vi "Process.vi"(8 "error in":errorcluster, 11 "MauiTemplate":refnum<class "SMO.UI.MAUI.Basic.lvclass">) -> (0 "error out":errorcluster, 3 "MauiTemplate out":refnum<class "SMO.UI.MAUI.Basic.lvclass">)   [LabVIEW 2016, in "SMO.UI.MAUI.Basic.lvclass"]
doc: "---------------------------------------------------------------\nJKI State Machine Objects™\nhttp://jki.net/state-machine-objects/\nCopyright (C) 2005-2015, JKI <info@jki.net>\nALL RIGHTS RESERVED"
uses:
  SMO.UI.MAUI.Basic.lvclass
  C:/Program Files (x86)/National Instruments/LabVIEW 2016/vi.lib/JKI/JKI SMO/SMO/SMO.lvclass
  C:/Program Files (x86)/National Instruments/LabVIEW 2016/vi.lib/Levylab/SMO.UI.MAUI/SMO.UI.MAUI.lvclass
  C:/Program Files (x86)/National Instruments/LabVIEW 2016/vi.lib/JKI/JKI SMO/SMO.UI/SMO.UI.lvclass
  <vilib>/JKI/JKI SMO/SMO/Typedefs/Parent Call--Enum.ctl
  <vilib>/Levylab/SMO.UI.MAUI/Typedefs/PanelData.ctl
  <vilib>/Levylab/SMO.UI.MAUI/SMO.UI.MAUI.lvclass
  <vilib>/JKI/JKI SMO/SMO/SMO.lvclass
  <vilib>/JKI/JKI SMO/SMO.UI/SMO.UI.lvclass
panel:
  out "Title":string
  in  "PopLeft":bool
  in  "PopRight":bool
  in  "Right Ring":u16(ring)
  in  "Left Ring":u16(ring)
  # "For instructions on how to use the JKI State Machine Objects, examples and video tutorials, visit:\nhttp://jki.net/state-machine-objects/\n\nJKI State Machine Objects™\nhttp://jki.net/state-machine-objects/\nCopyright (C) 2005-2015, JKI <info@jki.net>\nALL RIGHTS RESERVED"
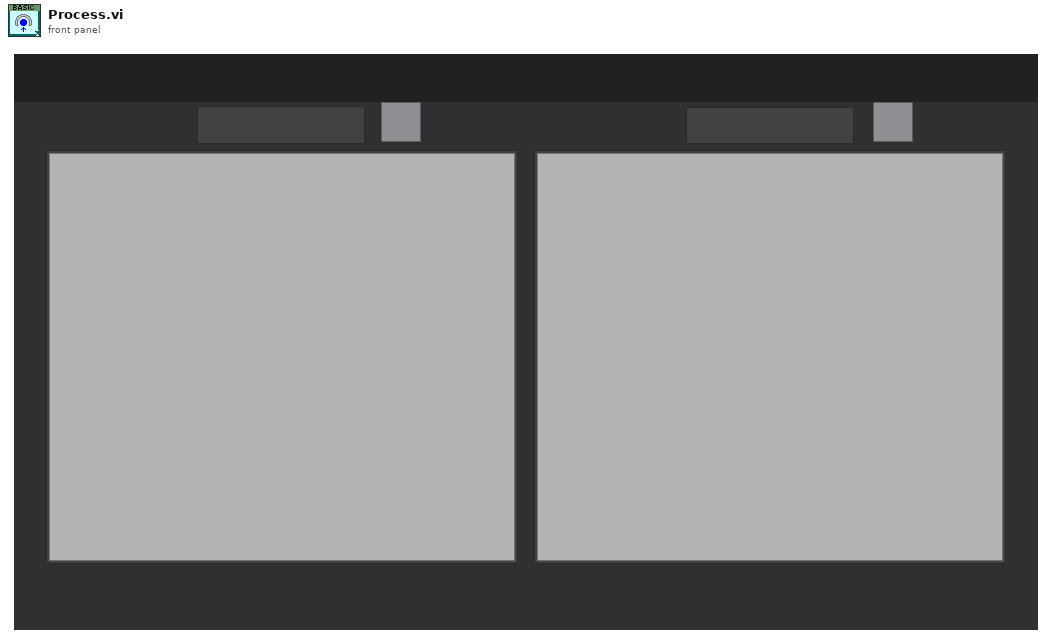
[diagram p1: front panel]
types:
  T1 = typedef "SMO.lvclass/Parent Call--Enum.ctl" = enum16{"Allows parent to run", "Does not request parent to run"}
  T2 = enum32{"invalid app kind", "Development System", "Run Time System", "Student Edition", "Embedded LabVIEW", "Evaluation", "Custom"}
  T3 = enum32{"Invalid", "Standard", "Closed", "Hidden", "Minimized", "Maximized"}
  T4 = enum32{"Bad", "Idle", "Run top level", "Running"}
  T5 = cluster{"Core":cluster{"Current VI Reference":refnum<vi>, "Close Panel on Exit?":bool, "error":errorcluster}, "MAUI":cluster{"Active Index":i32, "Panel Index":i32, "Pop Index":i32}, "Self Reference":refnum<class "SMO.UI.MAUI.Basic.lvclass">}
  T6 = cluster{"Active Index":i32, "Panel Index":i32, "Pop Index":i32}
  T7 = cluster{"Current VI Reference":refnum<vi>, "Close Panel on Exit?":bool, "error":errorcluster}
  T8 = typedef "SMO.lvclass/Protected Events.ctl" = cluster{"StopProcesses":refnum<user-event>, "AbortProcesses":refnum<user-event>, "Config Changed":refnum<user-event>, "Dependency":refnum<user-event>}
  T9 = typedef "SMO.UI.MAUI.lvclass/PublicEvents--Cluster.ctl" = cluster{"ReadyForInfo ":refnum<user-event>}
  T10 = typedef "SMO.UI.MAUI.lvclass/PanelData.ctl" = cluster{"SubPanel":refnum<vi>, "Ring":refnum<vi>, "Active":i32}
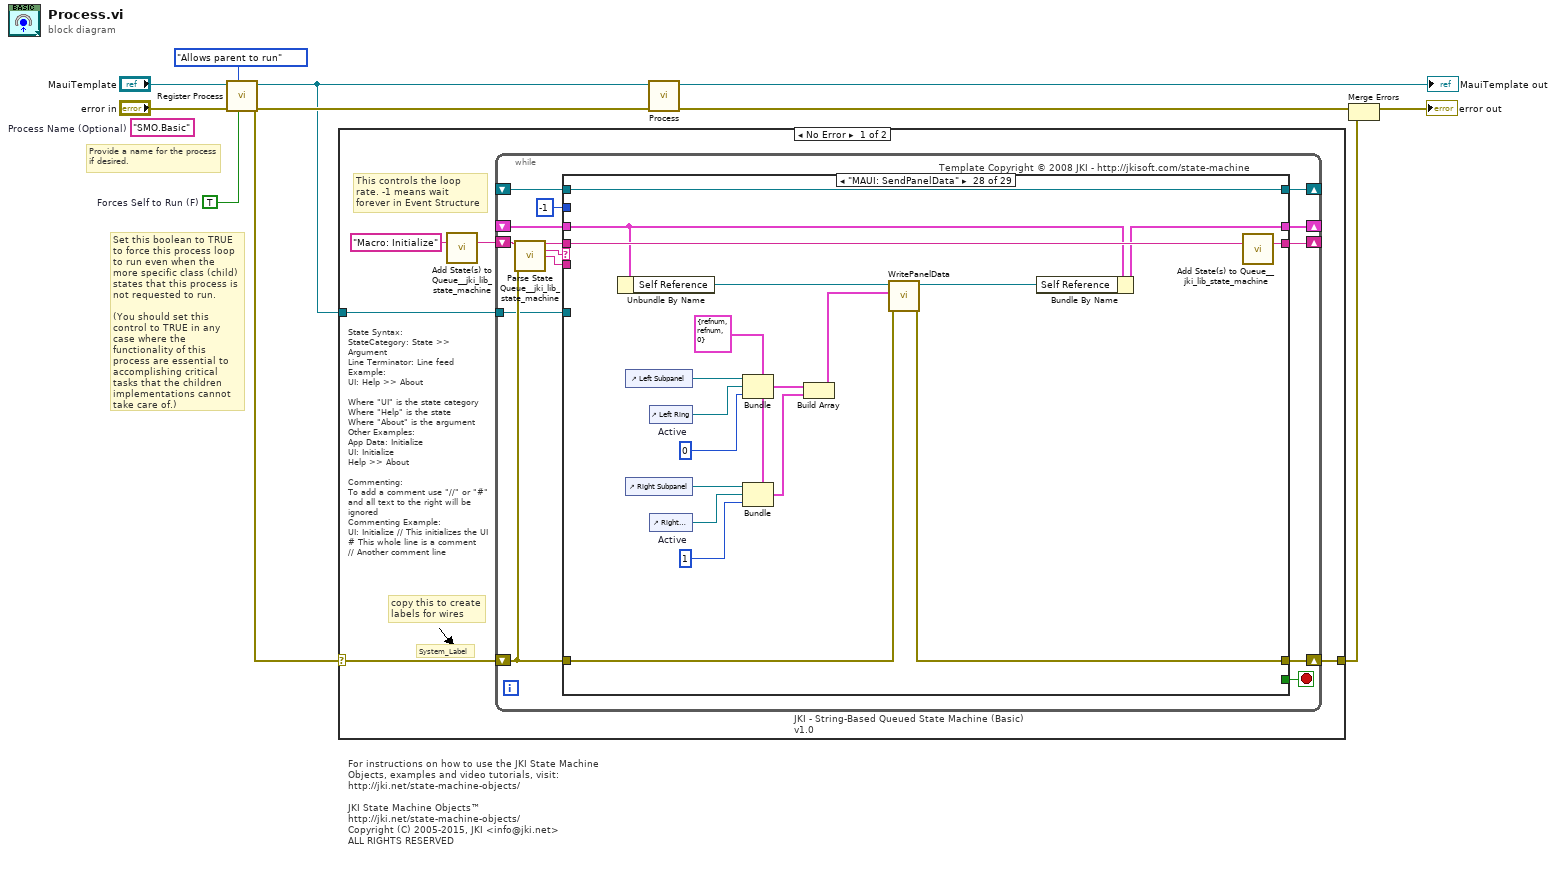
[diagram p0: block diagram]
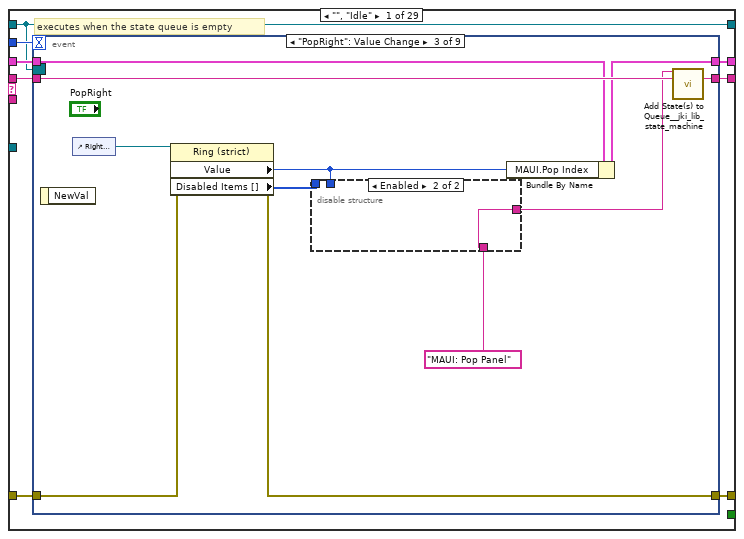
[diagram p2: hidden frame]
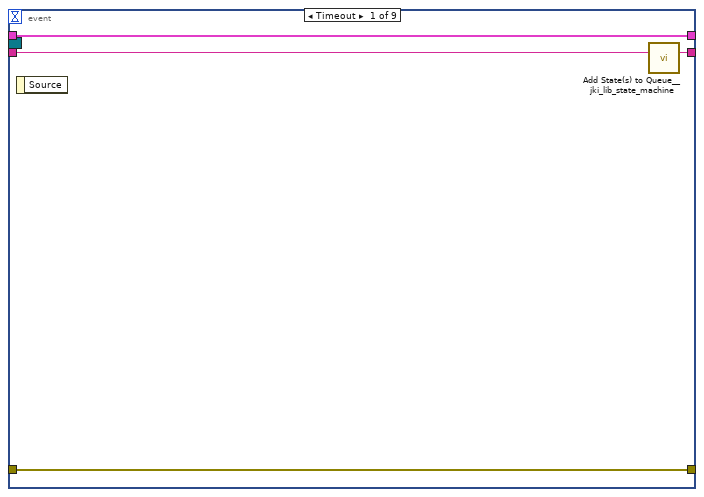
[diagram p3: hidden frame]
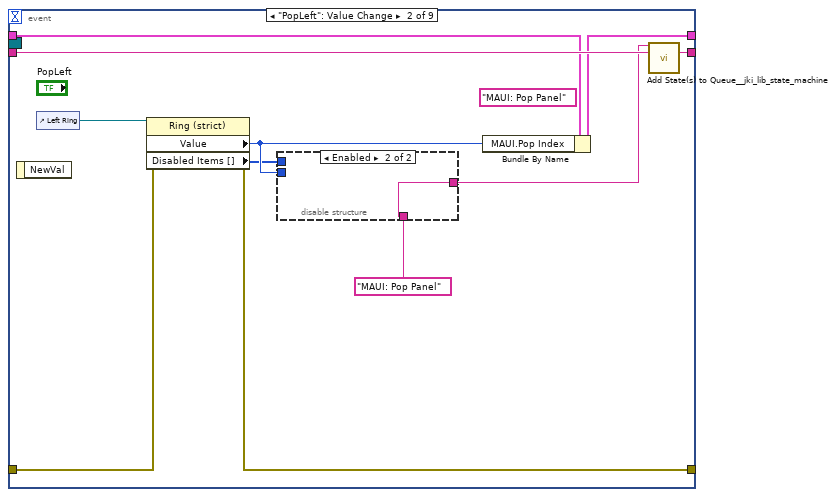
[diagram p4: hidden frame]
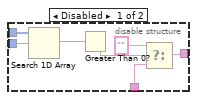
[diagram p5: hidden frame]
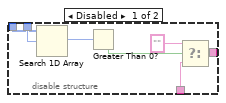
[diagram p6: hidden frame]
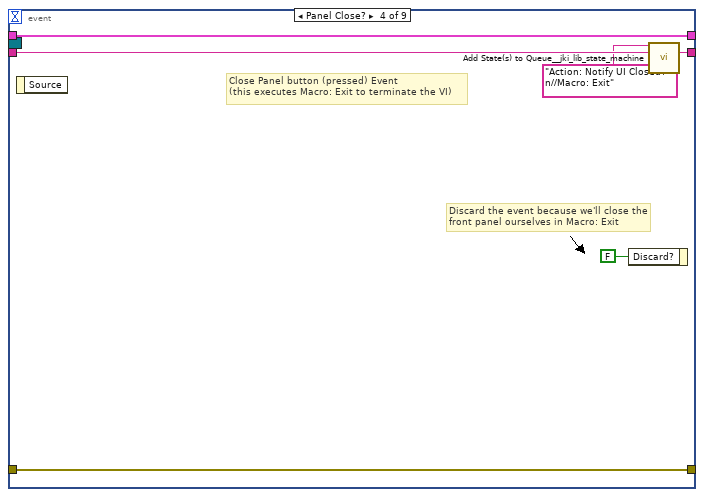
[diagram p7: hidden frame]
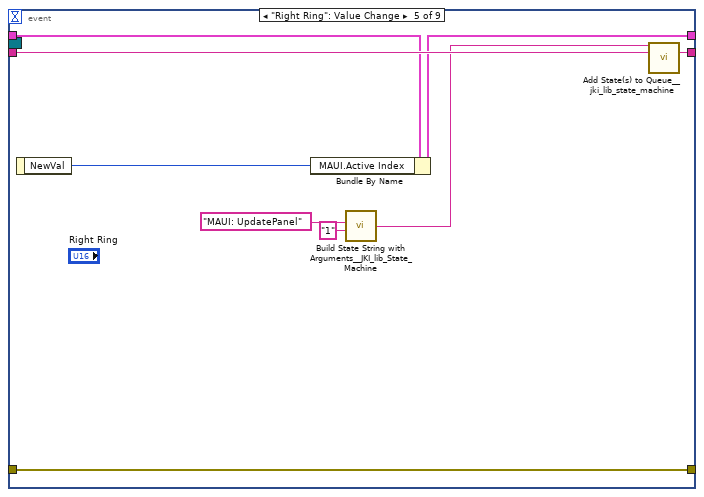
[diagram p8: hidden frame]
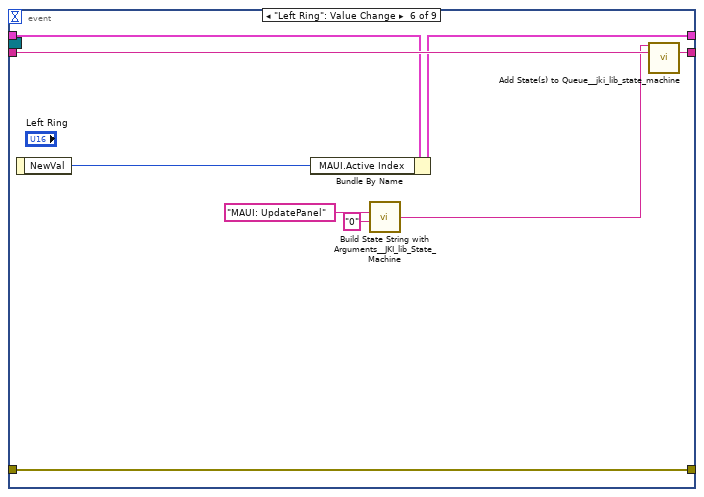
[diagram p9: hidden frame]
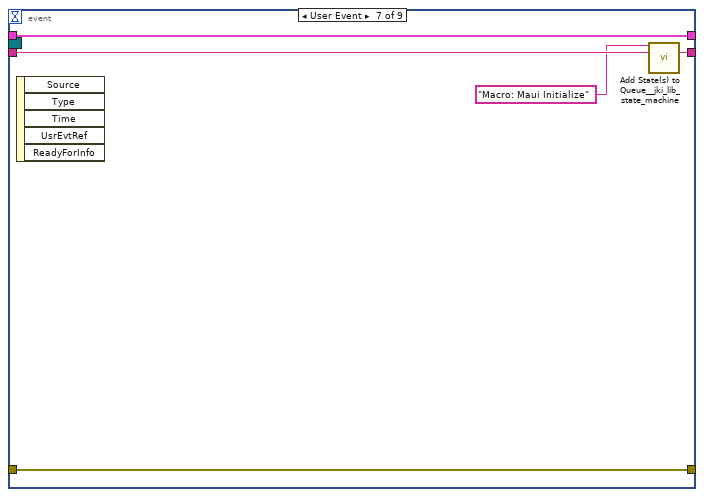
[diagram p10: hidden frame]
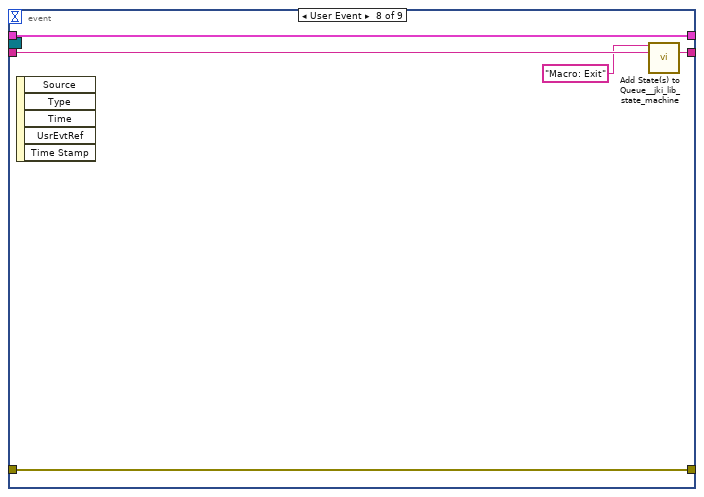
[diagram p11: hidden frame]
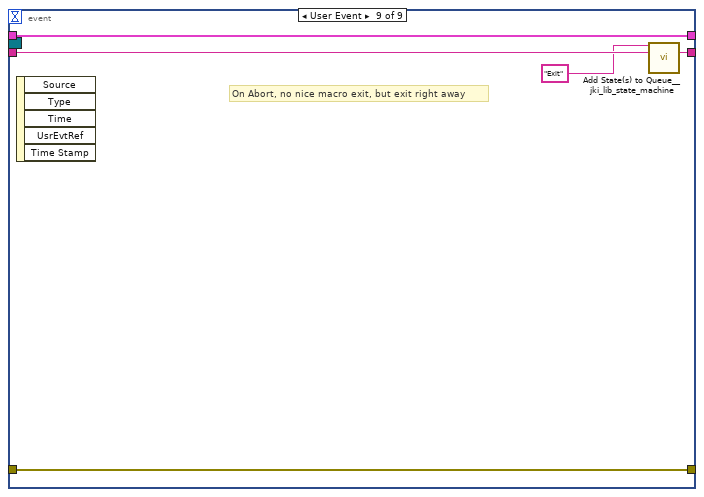
[diagram p12: hidden frame]
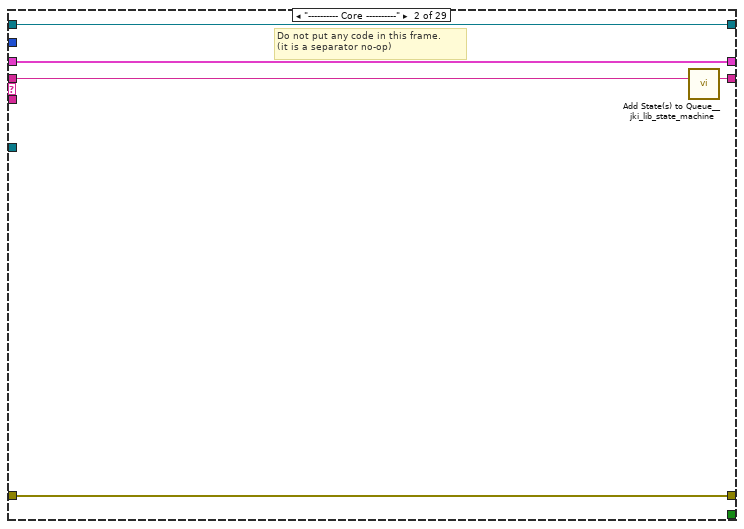
[diagram p13: hidden frame]
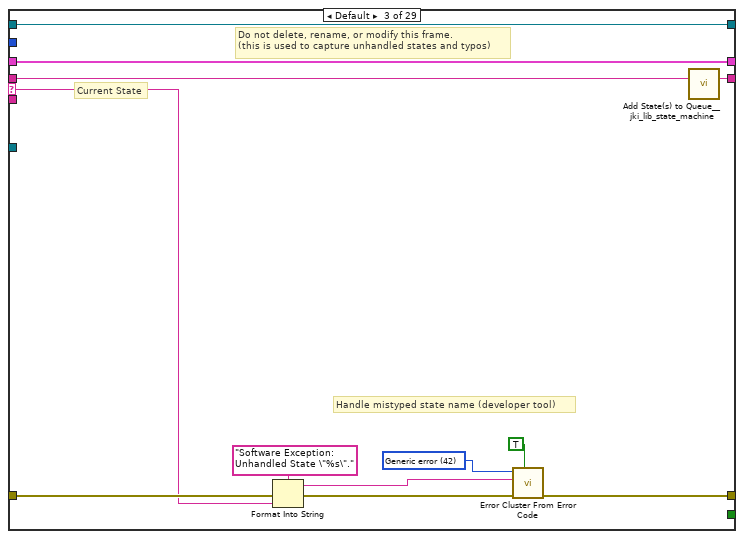
[diagram p14: hidden frame]
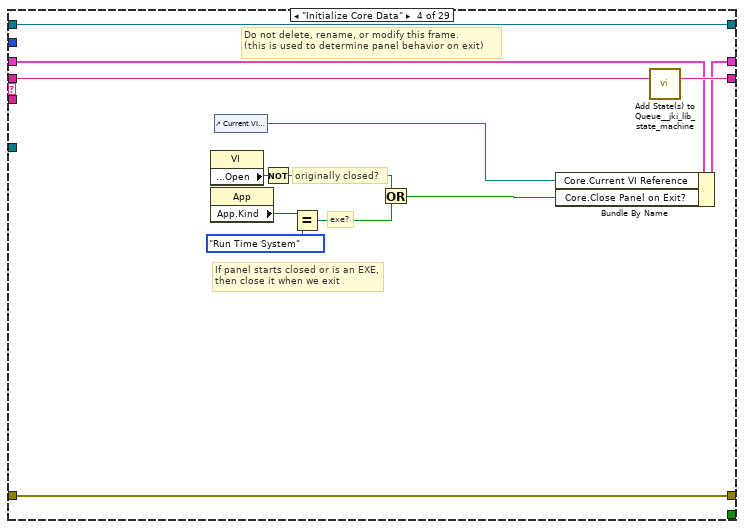
[diagram p15: hidden frame]
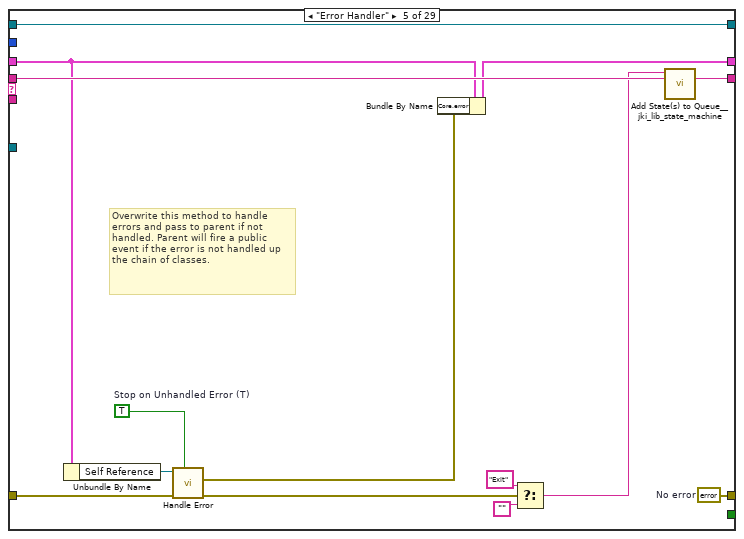
[diagram p16: hidden frame]
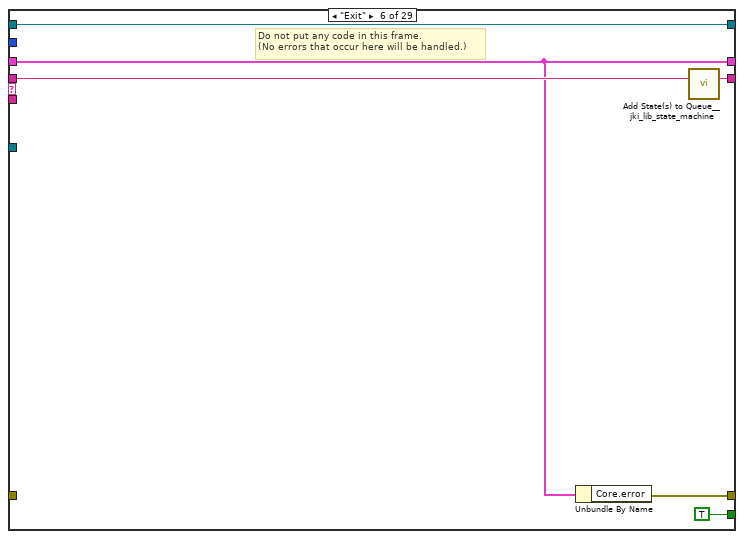
[diagram p17: hidden frame]
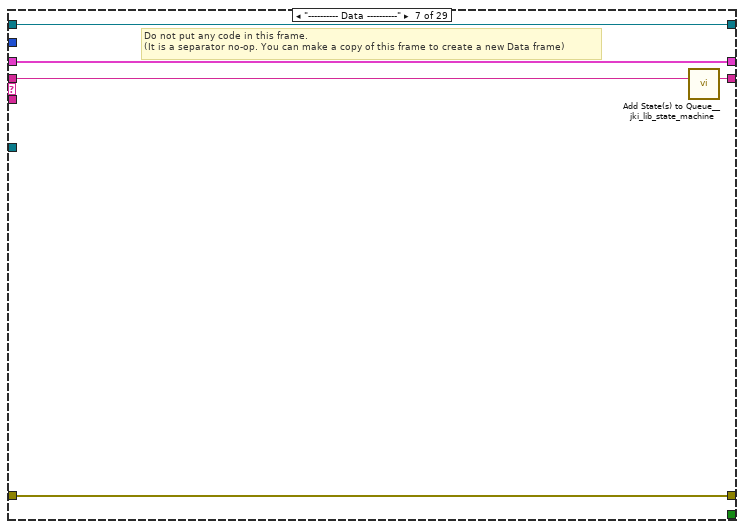
[diagram p18: hidden frame]
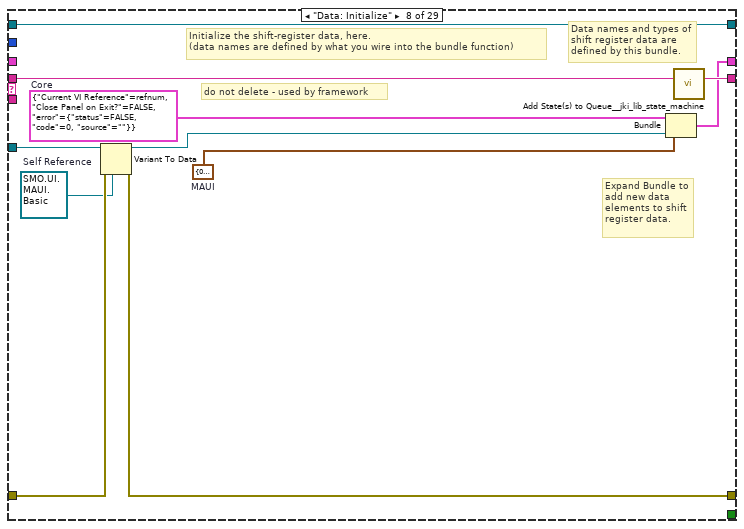
[diagram p19: hidden frame]
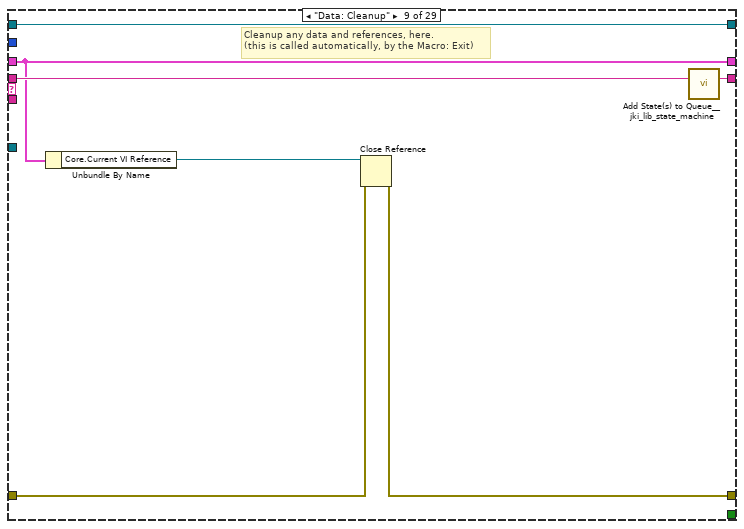
[diagram p20: hidden frame]
diagram:
  w2 = TRUE  # Forces Self to Run (F)
  (unwired) "SMO.Basic"  # Process Name (Optional)
  # "Provide a name for the process\nif desired."
  # "Set this boolean to TRUE to force this process loop to run even when the more specific class (child) states that this process is not requested to run.\n\n(You should set this control to TRUE in any case where the functionality of this process are essential to accomplishing critical tasks that the children implementations cannot take care of.)"
  # "For instructions on how to use the JKI State Machine Objects, examples and video tutorials, visit:\nhttp://jki.net/state-machine-objects/\n\nJKI State Machine Objects™\nhttp://jki.net/state-machine-objects/\nCopyright (C) 2005-2015, JKI <info@jki.net>\nALL RIGHTS RESERVED"
  n1 = call <vilib>:"Register Process.vi"("Forces Self to Run (F)"=w2, "Parent Call"=Parent_Call--Enum."Allows parent to run", "error in (no error)"="error in", "SMO"="MauiTemplate") -> ("error out"=w7:errorcluster, "SMO out"=w1:refnum<class "SMO.UI.MAUI.Basic.lvclass">)  [unwired: 6 in]
  n2 = case shown="No Error" w7 {
    selector: w7 -> [w12 w408]
    tunnel: w1 -> [w13 _]
    tunnel: [w11 w408] -> w4
    frame No Error {
      # "State Syntax:\nStateCategory: State >> Argument\nLine Terminator: Line feed\nExample:\nUI: Help >> About\n\nWhere \"UI\" is the state category\nWhere \"Help\" is the state\nWhere \"About\" is the argument\nOther Examples:\nApp Data: Initialize\nUI: Initialize\nHelp >> About\n\nCommenting:\nTo add a comment use \"//\" or \"#\" and all text to the right will be ignored\nCommenting Example:\nUI: Initialize // This initializes the UI\n# This whole line is a comment\n// Another comment line"
      # "copy this to create labels for wires"
      # "This controls the loop rate. -1 means wait forever in Event Structure"
      # "System_Label"
      n3 = call <vilib>:"Add State(s) to Queue__jki_lib_state_machine.vi"("State(s) in (\"\")"="Macro: Initialize") -> ("States Out"=w15:string)  [unwired: 14 in]
      n4 = while "JKI - String-Based Queued State Machine (Basic) v1.0" {
        shift-right: [w22] -> _
        shift-left: _ -> [w21]
        shift-right: [w25] -> w11
        shift-left: w12 -> [w19]
        shift-right: [w24] -> _
        shift-left: w15 -> [w26]
        tunnel: w13 -> [w18]
        shift-right: [w17] -> _
        shift-left: _ -> [w16]
        stop <- w23 stop-if-true
        # "Template Copyright © 2008 JKI - http://jkisoft.com/state-machine"
        n5 = call <vilib>:"Parse State Queue__jki_lib_state_machine.vi"("State Queue"=w26, "Error In (no error)"=w19) -> ("Remaining States"=w28:string, "Current State"=w29:string, "Arguments"=w27:string)  [unwired: 11 in]
        n6 = case shown="\"MAUI: SendPanelData\"" w29 {
          selector: w29 -> [_ _ w125 _ _ _ _ _ _ _ _ _ _ _ _ _ _ _ _ _ _ _ _ _ _ _ _ _ _]
          tunnel: w28 -> [w37 w123 w129 w148 w162 w168 w173 w184 w191 w196 w214 w221 w237 w269 w283 w289 w303 w308 w319 w324 w336 w342 w347 w354 w361 w366 w376 w395 w407]
          tunnel: w27 -> [_ _ _ _ _ _ _ _ _ _ _ w215 w231 _ _ _ _ _ _ _ _ _ _ _ _ _ _ _ w402]
          tunnel: w21 -> [w35 w120 w127 w139 w156 w164 w170 _ w186 w193 w209 w219 w233 w266 w279 w286 w294 w305 w316 w321 w334 w340 w345 w351 w357 w364 w371 w392 w404]
          tunnel: [w34 w121 w131 w145 w157 w163 w171 w180 w187 w194 w198 w216 w234 w267 w281 w287 w301 w306 w310 w322 w330 w338 w343 w348 w358 w362 w367 w379 w400] -> w25
          tunnel: w19 -> [w33 w121 w130 w145 w158 _ w171 w181 w188 w194 w204 w217 w235 w267 w281 w287 w301 w306 w311 w322 w331 w338 w343 w349 w358 w362 w368 w381 w401]
          tunnel: [w36 w122 w128 w147 w161 w167 w172 w183 w190 w195 w213 w220 w236 w268 w282 w288 w302 w307 w318 w323 w335 w341 w346 w353 w360 w365 w375 w394 w406] -> w24
          tunnel: [_ _ _ _ _ TRUE _ _ _ _ _ _ _ _ _ _ _ _ _ _ _ _ _ _ _ _ _ _ _] -> w23
          tunnel: [w32 w120 w127 w146 w155 w164 w170 w182 w186 w193 w208 w219 w233 w266 w279 w286 w294 w305 w316 w321 w334 w340 w345 w351 w356 w364 w370 w391 w403] -> w22
          tunnel: -1 ("Timeout") -> [w31 _ _ _ _ _ _ _ _ _ _ _ _ _ _ _ _ _ _ _ _ _ _ _ _ _ _ _ _]
          tunnel: w18 -> [_ _ _ _ _ _ _ w178 _ _ _ _ _ _ _ _ _ _ _ _ _ _ _ _ _ _ _ _ _]
          tunnel: [w30 w119 w124 w136 w160 w165 w169 w177 w185 w192 w212 w218 w230 w265 w280 w285 w295 w304 w317 w320 w333 w339 w344 w352 w359 w363 w374 w393 w405] -> w17
          tunnel: w16 -> [w30 w119 w124 w136 w160 w165 w169 w177 w185 w192 w212 w218 w230 w265 w280 w285 w295 w304 w317 w320 _ w339 w344 w352 w359 w363 w374 w393 w405]
          frame "", "Idle" {
            # "executes when the state queue is empty"
            n7 = event shown="[2] \"PopRight\": Value Change" {
              selector: w30 -> [_ _ _ _ _ _ _ _ _]
              dyn-events: _ -> [_ _ _ _ _ _ _ _ _]
              timeout: w31 -> [_ _ _ _ _ _ _ _ _]
              tunnel: w37 -> [w41 w52 w71 w85 w94 w103 w108 w113 w118]
              tunnel: [w40 w51 w70 w84 w93 w102 w107 w112 w117] -> w36
              tunnel: w35 -> [w39 w50 w69 w82 w91 w100 w106 w110 w115]
              tunnel: [w38 w47 w66 w83 w92 w101 w105 w111 w116] -> w34
              tunnel: w33 -> [w38 w48 w67 w83 w92 w101 w105 w111 w116]
              tunnel: [w39 w49 w68 w82 w90 w99 w106 w110 w115] -> w32
              event Timeout {
                n8 = event-data() -> ()  [unwired: 1 in, 1 out]
                n9 = call <vilib>:"Add State(s) to Queue__jki_lib_state_machine.vi"("State(s) in (\"\")"=w41) -> ("States Out"=w40:string)  [unwired: 14 in]
              }
              event "PopLeft": Value Change {
                (unwired) "MAUI: Pop Panel"
                n10 = event-data() -> ()  [unwired: 1 in, 1 out]
                n11 = control-ref of="Left Ring"() -> (w46:refnum<vi>)
                n12 = property class="Ring (strict)"(reference=w46, error in=w48) -> (error out=w47:errorcluster, "Value"=w45:u16, "Disabled Items []"=w44:i32[])  [unwired: 1 out]
                n13 = disable-structure shown="Enabled" {
                  disable-tunnel: w45 -> [w56 _]
                  disable-tunnel: w44 -> [w55 _]
                  disable-tunnel: "MAUI: Pop Panel" -> [w54 w60]
                  disable-tunnel: [w53 w60] -> w42
                  frame Disabled {
                    n14 = Search 1D Array(1D array=w55, element=w56) -> (index of element=w59:i32)  [unwired: 1 in]
                    n15 = Greater Than 0?(x=w59) -> (x > 0?=w57:bool)
                    n16 = Select(t="", s=w57, f=w54) -> (s? t:f=w53:string)
                  }
                  frame Enabled {
                  }
                }
                n17 = Bundle By Name(cluster=w50, "MAUI.Pop Index"=w45) -> (w49:T5)
                n18 = call <vilib>:"Add State(s) to Queue__jki_lib_state_machine.vi"("State(s) in Front (\"\")"=w42, "State(s) in (\"\")"=w52) -> ("States Out"=w51:string)  [unwired: 13 in]
              }
              event "PopRight": Value Change {
                n19 = event-data() -> ()  [unwired: 1 in, 1 out]
                n20 = control-ref of="Right Ring"() -> (w65:refnum<vi>)
                n21 = property class="Ring (strict)"(reference=w65, error in=w67) -> (error out=w66:errorcluster, "Value"=w64:u16, "Disabled Items []"=w63:i32[])  [unwired: 1 out]
                n22 = disable-structure shown="Enabled" {
                  disable-tunnel: w64 -> [w78 _]
                  disable-tunnel: w63 -> [w77 _]
                  disable-tunnel: "MAUI: Pop Panel" -> [w75 w79]
                  disable-tunnel: [w73 w79] -> w61
                  frame Disabled {
                    n23 = Search 1D Array(1D array=w77, element=w78) -> (index of element=w76:i32)  [unwired: 1 in]
                    n24 = Greater Than 0?(x=w76) -> (x > 0?=w72:bool)
                    n25 = Select(t="", s=w72, f=w75) -> (s? t:f=w73:string)
                  }
                  frame Enabled {
                  }
                }
                n26 = Bundle By Name(cluster=w69, "MAUI.Pop Index"=w64) -> (w68:T5)
                n27 = call <vilib>:"Add State(s) to Queue__jki_lib_state_machine.vi"("State(s) in Front (\"\")"=w61, "State(s) in (\"\")"=w71) -> ("States Out"=w70:string)  [unwired: 13 in]
              }
              event Panel Close? {
                # "Discard the event because we'll close the front panel ourselves in Macro: Exit"
                # "Close Panel button (pressed) Event\n(this executes Macro: Exit to terminate the VI)"
                n28 = event-data() -> ()  [unwired: 1 in, 1 out]
                n29 = event-data("Discard?"=FALSE) -> ()  [unwired: 1 in, 1 out]
                n30 = call <vilib>:"Add State(s) to Queue__jki_lib_state_machine.vi"("State(s) in Front (\"\")"="Action: Notify UI Closed\n//Macro: Exit", "State(s) in (\"\")"=w85) -> ("States Out"=w84:string)  [unwired: 13 in]
              }
              event "Right Ring": Value Change {
                n31 = event-data() -> ("NewVal"=w89:u16)  [unwired: 1 in]
                n32 = Bundle By Name(cluster=w91, "MAUI.Active Index"=w89) -> (w90:T5)
                n33 = call <vilib>:"Build State String with Arguments__JKI_lib_State_Machine.vi"("Arguments (\"\")"="1" ("Arguments (\"\")"), "State"="MAUI: UpdatePanel") -> ("State with Arguments"=w86:string)  [unwired: 4 in]
                n34 = call <vilib>:"Add State(s) to Queue__jki_lib_state_machine.vi"("State(s) in Front (\"\")"=w86, "State(s) in (\"\")"=w94) -> ("States Out"=w93:string)  [unwired: 13 in]
              }
              event "Left Ring": Value Change {
                n35 = event-data() -> ("NewVal"=w98:u16)  [unwired: 1 in]
                n36 = Bundle By Name(cluster=w100, "MAUI.Active Index"=w98) -> (w99:T5)
                n37 = call <vilib>:"Build State String with Arguments__JKI_lib_State_Machine.vi"("Arguments (\"\")"="0" ("Arguments (\"\")"), "State"="MAUI: UpdatePanel") -> ("State with Arguments"=w95:string)  [unwired: 4 in]
                n38 = call <vilib>:"Add State(s) to Queue__jki_lib_state_machine.vi"("State(s) in Front (\"\")"=w95, "State(s) in (\"\")"=w103) -> ("States Out"=w102:string)  [unwired: 13 in]
              }
              event User Event {
                n39 = event-data() -> ()  [unwired: 1 in, 5 out]
                n40 = call <vilib>:"Add State(s) to Queue__jki_lib_state_machine.vi"("State(s) in Front (\"\")"="Macro: Maui Initialize", "State(s) in (\"\")"=w108) -> ("States Out"=w107:string)  [unwired: 13 in]
              }
              event User Event {
                n41 = event-data() -> ()  [unwired: 1 in, 5 out]
                n42 = call <vilib>:"Add State(s) to Queue__jki_lib_state_machine.vi"("State(s) in Front (\"\")"="Macro: Exit", "State(s) in (\"\")"=w113) -> ("States Out"=w112:string)  [unwired: 13 in]
              }
              event User Event {
                # "On Abort, no nice macro exit, but exit right away"
                n43 = event-data() -> ()  [unwired: 1 in, 5 out]
                n44 = call <vilib>:"Add State(s) to Queue__jki_lib_state_machine.vi"("State(s) in Front (\"\")"="Exit", "State(s) in (\"\")"=w118) -> ("States Out"=w117:string)  [unwired: 13 in]
              }
            }
          }
          frame "---------- Core ----------" {
            # "Do not put any code in this frame.\n(it is a separator no-op)"
            n45 = call <vilib>:"Add State(s) to Queue__jki_lib_state_machine.vi"("State(s) in (\"\")"=w123) -> ("States Out"=w122:string)  [unwired: 14 in]
          }
          frame Default {
            w134 = 42 items=["No error", "Argument error", "Memory is full", "Out of zone", "End of file", "File already open", "Generic file I/O error", "File not found", "File permission error", "Disk is full", "Duplicate path", "Too many files open", "System feature not enabled", "Resource file not found", "Cannot add resource", "Resource not found", "Image not found", "Image memory error", "Pen does not exist", "Config type invalid", "Config token not found", "Config parse error", "Config memory error", "Bad external code format", "Bad external code offset", "External code not present", "Null window", "Destroy window error", "Null menu", "Print aborted", "Bad print record", "Print driver error", "Windows error during printing", "Memory error during printing", "Print dialog error", "Generic print error", "Invalid device refnum", "Device not found", "Device parameter error", "Device unit error", "Cannot open device", "Device call aborted", "Generic error", "Cancelled by user", "Object ID too low", "Object ID too high", "Object not in heap", "Unknown heap", "Unknown object (invalid DefProc)", "Unknown object (DefProc not in table)", "Message out of range", "Invalid (null) method", "Unknown message", "Manager call not supported", "Bad address", "Network operation in progress", "Network operation timed out", "Connection is busy", "Network attribute not supported", "Network error", "Address in use", "System out of memory", "Connection aborted", "Connection refused", "Not connected", "Already connected", "Connection closed", "Initialization error (interapplication manager)", "Bad occurrence", "Wait on unbound occurrence handler", "Occurrence queue overflow", "Datalog type conflict", "Unused", "Unrecognized type (interapplication manager)", "Memory corrupt", "Failed to make temporary DLL", "Old CIN version", "Drag socket not found", "Failed to load drop-object", "Failed to register OLE object", "Failed to release OLE object", "Format specifier type mismatch", "Unknown format specifier", "Too few format specifiers", "Too many format specifiers", "Scan failed", "Newer CIN version", "Error converting to variant", "Runtime menu error", "Password tampered", "Variant attribute not found", "Incompatible variant data type", "Event data is not available", "Event Store is not present", "Occurrence is not found", "Event Queue is not created", "Event info is not available", "Refnum passed is NULL", "Error retrieving Class GUID", "Error retrieving CoClass GUID", "Error retrieving TypeLib GUID.", "Bad built application magic bytes.", "Specific driver is different from the specific driver associated with the Logical Name.", "There is no session opened to the class driver.", "Max Error", "MAX - Error with config objects", "MAX - Error loading configuration", "MAX - Group not supported"]
            # "Current State"
            # "Do not delete, rename, or modify this frame.\n(this is used to capture unhandled states and typos)"
            # "Handle mistyped state name (developer tool)"
            n46 = Format Into String(format string="Software Exception: Unhandled State \"%s\"." ("message"), error in=w130, w125) -> (resulting string=w133:string, error out=w132:errorcluster)  [unwired: 1 in]
            n47 = call <vilib>:"Error Cluster From Error Code.vi"("show call chain? (False)"=TRUE, "error in (no error)"=w132, "error message (\"\")"=w133, "error code (0)"=w134) -> ("error out"=w131:errorcluster)  [unwired: 5 in]
            n48 = call <vilib>:"Add State(s) to Queue__jki_lib_state_machine.vi"("State(s) in (\"\")"=w129) -> ("States Out"=w128:string)  [unwired: 14 in]
          }
          frame "Initialize Core Data" {
            # "Do not delete, rename, or modify this frame.\n(this is used to determine panel behavior on exit)"
            # "originally closed?"
            # "exe?"
            # "If panel starts closed or is an EXE, then close it when we exit"
            n49 = property class="VI"() -> ("Front Panel.Open"=w144:bool)  [unwired: 2 in, 2 out]
            n50 = property class="App"() -> ("App.Kind"=w143:T2)  [unwired: 2 in, 2 out]
            n51 = control-ref of="Current VI Reference"() -> (w137:refnum<vi>)
            n52 = Not(x=w144) -> (.not. x?=w141:bool)
            n53 = Equal?(x=w143, y=T2."Run Time System" ("Application:Kind")) -> (x = y?=w140:bool)
            n54 = Or(x=w141, y=w140) -> (x .or. y?=w138:bool)
            n55 = Bundle By Name(cluster=w139, "Core.Current VI Reference"=w137, "Core.Close Panel on Exit?"=w138) -> (w146:T5)
            n56 = call <vilib>:"Add State(s) to Queue__jki_lib_state_machine.vi"("State(s) in (\"\")"=w148) -> ("States Out"=w147:string)  [unwired: 14 in]
          }
          frame "Error Handler" {
            w149 = TRUE  # Stop on Unhandled Error (T)
            w157 = errorcluster {"status"=FALSE, "code"=0, "source"=""}  # No error
            # "Overwrite this method to handle errors and pass to parent if not handled. Parent will fire a public event if the error is not handled up the chain of classes."
            n57 = Unbundle By Name(w156) -> ("Self Reference"=w159:refnum<class "SMO.UI.MAUI.Basic.lvclass">)
            n58 = call-dynamic "Handle Error.vi"("Stop on Unhandled Error (T)"=w149, "error in"=w158, "SMO"=w159) -> ("handling error"=w150:errorcluster, "Unhandled error"=w153:errorcluster)  [unwired: 6 in, 1 out]
            n59 = Bundle By Name(cluster=w156, "Core.error"=w153) -> (w155:T5)
            n60 = Select(t="Exit", s=w150, f="") -> (s? t:f=w154:string)
            n61 = call <vilib>:"Add State(s) to Queue__jki_lib_state_machine.vi"("State(s) in Front (\"\")"=w154, "State(s) in (\"\")"=w162) -> ("States Out"=w161:string)  [unwired: 13 in]
          }
          frame "Exit" {
            # "Do not put any code in this frame.\n(No errors that occur here will be handled.)"
            n62 = Unbundle By Name(w164) -> ("Core.error"=w163:errorcluster)
            n63 = call <vilib>:"Add State(s) to Queue__jki_lib_state_machine.vi"("State(s) in (\"\")"=w168) -> ("States Out"=w167:string)  [unwired: 14 in]
          }
          frame "---------- Data ----------" {
            # "Do not put any code in this frame.\n(It is a separator no-op. You can make a copy of this frame to create a new Data frame)"
            n64 = call <vilib>:"Add State(s) to Queue__jki_lib_state_machine.vi"("State(s) in (\"\")"=w173) -> ("States Out"=w172:string)  [unwired: 14 in]
          }
          frame "Data: Initialize" {
            w175 = T6 {"Active Index"=0, "Panel Index"=1, "Pop Index"=1}  # MAUI
            w176 = T7 {"Current VI Reference"=refnum, "Close Panel on Exit?"=FALSE, "error"={"status"=FALSE, "code"=0, "source"=""}}  # Core
            w179 = refnum<class "SMO.UI.MAUI.Basic.lvclass"> refnum  # Self Reference
            # "do not delete - used by framework"
            # "Expand Bundle to add new data elements to shift register data."
            # "Data names and types of shift register data are defined by this bundle."
            # "Initialize the shift-register data, here.\n(data names are defined by what you wire into the bundle function)"
            n65 = Variant To Data(error in=w181, type=w179, Variant=w178) -> (data=w174:refnum<class "SMO.UI.MAUI.Basic.lvclass">, error out=w180:errorcluster)
            n66 = Bundle("Core"=w176, "MAUI"=w175, "Self Reference"=w174) -> (w182:T5)  [unwired: 1 in]
            n67 = call <vilib>:"Add State(s) to Queue__jki_lib_state_machine.vi"("State(s) in (\"\")"=w184) -> ("States Out"=w183:string)  [unwired: 14 in]
          }
          frame "Data: Cleanup" {
            # "Cleanup any data and references, here.\n(this is called automatically, by the Macro: Exit)"
            n68 = Unbundle By Name(w186) -> ("Core.Current VI Reference"=w189:refnum<vi>)
            n69 = Close Reference(reference=w189, error in (no error)=w188) -> (error out=w187:errorcluster)
            n70 = call <vilib>:"Add State(s) to Queue__jki_lib_state_machine.vi"("State(s) in (\"\")"=w191) -> ("States Out"=w190:string)  [unwired: 14 in]
          }
          frame "---------- UI ----------" {
            # "Do not put any code in this frame.\n(It is a separator no-op. You can make a copy of this frame to create a new UI frame)"
            n71 = call <vilib>:"Add State(s) to Queue__jki_lib_state_machine.vi"("State(s) in (\"\")"=w196) -> ("States Out"=w195:string)  [unwired: 14 in]
          }
          frame "UI: Initialize" {
            # "Initialize the User Interface, here.\n(this is called automatically, by the Macro: Init)"
            n72 = control-ref of="Right Ring"() -> (w211:refnum<vi>)
            n73 = control-ref of="Left Ring"() -> (w206:refnum<vi>)
            n74 = property class="Ring (strict)"(reference=w211, error in=w204, "Value"=u16 1) -> (error out=w202:errorcluster)  [unwired: 1 out]
            n75 = property class="Ring (strict)"(reference=w206, error in=w204, "Value"=u16 0) -> (error out=w203:errorcluster)  [unwired: 1 out]
            n76 = Unbundle By Name(w209) -> ("Self Reference"=w201:refnum<class "SMO.UI.MAUI.Basic.lvclass">, "Core.Current VI Reference"=w200:refnum<vi>)
            n77 = Merge Errors(w202, w203) -> (w199:errorcluster)
            n78 = call <vilib>:"ArrangeFrontPanel.vi"("error in (no error)"=w199, "This VI"=w200, "MAUI in"=w201) -> ("error out"=w198:errorcluster, "MAUI out"=w197:refnum<class "SMO.UI.MAUI.Basic.lvclass">)  [unwired: 7 in]
            n79 = Bundle By Name(cluster=w209, "Self Reference"=w197) -> (w208:T5)
            n80 = call <vilib>:"Add State(s) to Queue__jki_lib_state_machine.vi"("State(s) in (\"\")"=w214) -> ("States Out"=w213:string)  [unwired: 14 in]
            "Title" <- "Generic" ("Title")
          }
          frame "UI: Cursor Set" {
            # "Argument"
            # "Initialize the User Interface, here.\n(this is called automatically, by the Macro: Init)"
            n81 = disable-structure shown="Default" {
              disable-tunnel: w217 -> [w222 w225]
              disable-tunnel: [w222 w224] -> w216
              disable-tunnel: w215 -> [_ w223]
              frame condition #0 {
              }
              frame condition #1 (active) {
                n82 = case shown="\"Idle\", Default" w223 {
                  tunnel: w225 -> [w227 w229]
                  tunnel: [w226 w228] -> w224
                  frame "Idle", Default {
                    n83 = call <vilib>:"Unset Busy.vi"("error in (no error)"=w227) -> ("error out"=w226:errorcluster)  [unwired: 10 in]
                  }
                  frame "Busy" {
                    n84 = call <vilib>:"Set Busy.vi"("error in (no error)"=w229) -> ("error out"=w228:errorcluster)  [unwired: 9 in, 1 out]
                  }
                }
              }
            }
            n85 = call <vilib>:"Add State(s) to Queue__jki_lib_state_machine.vi"("State(s) in (\"\")"=w221) -> ("States Out"=w220:string)  [unwired: 14 in]
          }
          frame "UI: Front Panel State" {
            # "Argument"
            # "Set Front Panel Open or Closed\n(Usage: \"UI: Front Panel State >> Open|Close\")"
            n86 = Unbundle By Name(w233) -> ("Core.Current VI Reference"=w232:refnum<vi>)
            n87 = disable-structure shown="Default" {
              disable-tunnel: w235 -> [w241 w264]
              disable-tunnel: [w240 w264] -> w234
              disable-tunnel: w232 -> [w239 _]
              disable-tunnel: w231 -> [w238 _]
              frame condition #0 (active) {
                n88 = case shown="\"Close\"" w238 {
                  tunnel: w241 -> [w245 w258]
                  tunnel: [w247 w259] -> w240
                  tunnel: w239 -> [w246 w256]
                  frame "Open", Default {
                    n89 = property class="VI"(reference=w246, error in=w245) -> (reference out=w243:refnum<vi>, error out=w244:errorcluster, "FP.State"=w242:T3)
                    n90 = case shown="\"Closed\"" w242 {
                      tunnel: [w250 w253] -> w247
                      tunnel: w244 -> [w249 w253]
                      tunnel: w243 -> [w248 _]
                      frame "Closed" {
                        n91 = invoke class="VI" method="FP.Open"(reference=w248, error in=w249, "Activate"=TRUE, "State"=T3."Standard") -> (error out=w250:errorcluster)  [unwired: 1 in, 4 out]
                      }
                      frame Default {
                      }
                    }
                  }
                  frame "Close" {
                    n92 = property class="VI"(reference=w256, error in=w258) -> (reference out=w255:refnum<vi>, error out=w257:errorcluster, "FP.State"=w254:T3)
                    n93 = case shown="Default" w254 {
                      tunnel: [w260 w263] -> w259
                      tunnel: w257 -> [w260 w262]
                      tunnel: w255 -> [_ w261]
                      frame "Invalid", "Closed" {
                      }
                      frame Default {
                        n94 = invoke class="VI" method="FP.Close"(reference=w261, error in=w262) -> (error out=w263:errorcluster)  [unwired: 1 in, 2 out]
                      }
                    }
                  }
                }
              }
              frame condition #1 {
              }
            }
            n95 = call <vilib>:"Add State(s) to Queue__jki_lib_state_machine.vi"("State(s) in (\"\")"=w237) -> ("States Out"=w236:string)  [unwired: 14 in]
          }
          frame "---------- Macro ----------" {
            # "Do not put any code in this frame.\n(It is a separator no-op. You can make a copy of this frame to create a new Macro frame)"
            n96 = call <vilib>:"Add State(s) to Queue__jki_lib_state_machine.vi"("State(s) in (\"\")"=w269) -> ("States Out"=w268:string)  [unwired: 14 in]
          }
          frame "Macro: Initialize" {
            w274 = "UI: Initialize\nUI: Front Panel State >> Open"  # UI: Initialize UI: Front Panel State >> Open
            w270 = "Process: Sync"
            # "Initialization Macro\n(This is called once, when the VI starts)"
            n97 = control-ref of="This VI"() -> (w272:refnum<vi>)
            n98 = property class="VI"(reference=w272) -> ("Exec.State"=w271:T4)  [unwired: 1 in, 2 out]
            n99 = Equal?(x=w271, y=T4."Run top level") -> (x = y?=w277:bool)
            n100 = Select(t=w270, s=w277, f="") -> ()  [unwired: 1 out]
            n101 = call <vilib>:"Add State(s) to Queue__jki_lib_state_machine.vi"("State(s) in Front (\"\")"="Data: Initialize\nInitialize Core Data\nEvents: Register", "State(s) in (\"\")"=w270, "State(s) at Back (\"\")"=w274) -> ("States Out"=w273:string)  [unwired: 12 in]
            n102 = call <vilib>:"Add State(s) to Queue__jki_lib_state_machine.vi"("State(s) in Front (\"\")"=w273, "State(s) in (\"\")"=w283) -> ("States Out"=w282:string)  [unwired: 13 in]
          }
          frame "Macro: Maui Initialize" {
            # "Do not put any code in this frame.\n(It is a separator no-op. You can make a copy of this frame to create a new Macro frame)"
            n103 = call <vilib>:"Add State(s) to Queue__jki_lib_state_machine.vi"("State(s) in Front (\"\")"="MAUI: SendPanelData", "State(s) in (\"\")"=w289) -> ("States Out"=w288:string)  [unwired: 13 in]
          }
          frame "Macro: Exit" {
            # "Exit Macro\n(This is called once, when the VI exits)"
            n104 = Unbundle By Name(w294) -> ("Core.Close Panel on Exit?"=w300:bool)
            n105 = Select(t="UI: Front Panel State >> Close", s=w300, f="") -> (s? t:f=w297:string)
            n106 = call <vilib>:"Add State(s) to Queue__jki_lib_state_machine.vi"("State(s) in Front (\"\")"="Data: Cleanup\nEvents: Unregister", "State(s) in (\"\")"="Process: Sync", "State(s) at Back (\"\")"="Exit") -> ("States Out"=w291:string)  [unwired: 12 in]
            n107 = call <vilib>:"Add State(s) to Queue__jki_lib_state_machine.vi"("State(s) in (\"\")"=w297, "State(s) at Back (\"\")"=w291) -> ("States Out"=w296:string)  [unwired: 13 in]
            n108 = call <vilib>:"Add State(s) to Queue__jki_lib_state_machine.vi"("State(s) in Front (\"\")"=w296, "State(s) in (\"\")"=w303) -> ("States Out"=w302:string)  [unwired: 13 in]
          }
          frame "---------- Process ----------" {
            # "Template Separator\n(You can make a copy of, or modify, this frame)"
            n109 = call <vilib>:"Add State(s) to Queue__jki_lib_state_machine.vi"("State(s) in (\"\")"=w308) -> ("States Out"=w307:string)  [unwired: 14 in]
          }
          frame "Process: Sync" {
            n110 = Unbundle By Name(w316) -> ("Self Reference"=w312:refnum<class "SMO.UI.MAUI.Basic.lvclass">)
            n111 = call <vilib>:"WaitOnProcessSync.vi"("error in (no error)"=w311, "SMO"=w312) -> ("error out"=w310:errorcluster, "Don't run?"=w315:bool)  [unwired: 7 in, 1 out]
            n112 = Select(t="Data: Cleanup\nEvents: Unregister\nExit", s=w315, f="") -> (s? t:f=w309:string)
            n113 = call <vilib>:"Add State(s) to Queue__jki_lib_state_machine.vi"("State(s) in Front (\"\")"=w309, "State(s) in (\"\")"=w319) -> ("States Out"=w318:string)  [unwired: 13 in]
          }
          frame "---------- Events ----------" {
            # "Template Separator\n(You can make a copy of, or modify, this frame)"
            n114 = call <vilib>:"Add State(s) to Queue__jki_lib_state_machine.vi"("State(s) in (\"\")"=w324) -> ("States Out"=w323:string)  [unwired: 14 in]
          }
          frame "Events: Register" {
            # "Expand to add\nmore events"
            n115 = Unbundle By Name(w334) -> ("Self Reference"=w327:refnum<class "SMO.UI.MAUI.Basic.lvclass">)
            n116 = call <vilib>:"GetProtectedEvents.vi"("SMO"=w327) -> ("error out"=w328:errorcluster, "SMO Protected Events"=w332:T8)  [unwired: 8 in, 1 out]
            n117 = call <vilib>:"SMO.UI.MAUI.GetPublicEvents.vi"("MAUI"=w327) -> ("error out"=w326:errorcluster, "Public Events"=w325:T9)  [unwired: 8 in, 1 out]
            n118 = register-events(w332, w325) -> (reference out=w333:refnum<event-registration>, error out=w329:errorcluster)  [unwired: 2 in]
            n119 = Merge Errors(w331, w329, w328, w326) -> (w330:errorcluster)
            n120 = call <vilib>:"Add State(s) to Queue__jki_lib_state_machine.vi"("State(s) in (\"\")"=w336) -> ("States Out"=w335:string)  [unwired: 14 in]
          }
          frame "Events: Unregister" {
            n121 = Unregister For Events(event registration refnum=w339, error in=w338) -> (error out=w337:errorcluster)
            n122 = call <vilib>:"Clear Errors.vi"("error in (no error)"=w337) -> ()  [unwired: 5 in, 2 out]
            n123 = call <vilib>:"Add State(s) to Queue__jki_lib_state_machine.vi"("State(s) in (\"\")"=w342) -> ("States Out"=w341:string)  [unwired: 14 in]
          }
          frame "---------- Action ----------" {
            n124 = call <vilib>:"Add State(s) to Queue__jki_lib_state_machine.vi"("State(s) in (\"\")"=w347) -> ("States Out"=w346:string)  [unwired: 14 in]
          }
          frame "Action: Notify UI Closed" {
            n125 = Unbundle By Name(w351) -> ("Self Reference"=w350:refnum<class "SMO.UI.MAUI.Basic.lvclass">)
            n126 = call <vilib>:"Hide.vi"("error in (no error)"=w349, "SMO.UI"=w350) -> ("error out"=w348:errorcluster)  [unwired: 8 in, 1 out]
            n127 = call <vilib>:"Add State(s) to Queue__jki_lib_state_machine.vi"("State(s) in (\"\")"=w354) -> ("States Out"=w353:string)  [unwired: 14 in]
          }
          frame "Action: Template" {
            n128 = Unbundle By Name(w357) -> ("Self Reference"=w355:refnum<class "SMO.UI.MAUI.Basic.lvclass">)
            n129 = Bundle By Name(cluster=w357, "Self Reference"=w355) -> (w356:T5)
            n130 = call <vilib>:"Add State(s) to Queue__jki_lib_state_machine.vi"("State(s) in (\"\")"=w361) -> ("States Out"=w360:string)  [unwired: 14 in]
          }
          frame "---------- MAUI ----------" {
            # "Left Subpanel is index 0\nRight Subpanel is Index 1"
            n131 = call <vilib>:"Add State(s) to Queue__jki_lib_state_machine.vi"("State(s) in (\"\")"=w366) -> ("States Out"=w365:string)  [unwired: 14 in]
          }
          frame "MAUI: Pop Panel" {
            # "Left Subpanel is index 0\nRight Subpanel is Index 1"
            n132 = Unbundle By Name(w371) -> ("Self Reference"=w373:refnum<class "SMO.UI.MAUI.Basic.lvclass">, "MAUI.Pop Index"=w372:i32)
            n133 = call <vilib>:"PopSubpanel.vi"("error in (no error)"=w368, "Pop Index"=w372, "SMO.UI.MAUI in"=w373) -> ("error out"=w367:errorcluster, "SMO.UI.MAUI out"=w369:refnum<class "SMO.UI.MAUI.Basic.lvclass">)  [unwired: 7 in]
            n134 = Bundle By Name(cluster=w371, "Self Reference"=w369) -> (w370:T5)
            n135 = call <vilib>:"Add State(s) to Queue__jki_lib_state_machine.vi"("State(s) in (\"\")"=w376) -> ("States Out"=w375:string)  [unwired: 14 in]
          }
          frame "MAUI: SendPanelData" {
            w384 = T10 {"SubPanel"=refnum, "Ring"=refnum, "Active"=0} ("Panel")
            w386 = 1  # Active
            w388 = 0  # Active
            n136 = Unbundle By Name(w392) -> ("Self Reference"=w383:refnum<class "SMO.UI.MAUI.Basic.lvclass">)
            n137 = control-ref of="Left Subpanel"() -> (w378:refnum<vi>)
            n138 = control-ref of="Right Subpanel"() -> (w377:refnum<vi>)
            n139 = control-ref of="Left Ring"() -> (w389:refnum<vi>)
            n140 = control-ref of="Right Ring"() -> (w387:refnum<vi>)
            n141 = Bundle(cluster=w384, "SubPanel"=w378, "Ring"=w389, "Active"=w388) -> (w390:T10)
            n142 = Bundle(cluster=w384, "SubPanel"=w377, "Ring"=w387, "Active"=w386) -> (w385:T10)
            n143 = Build Array(w390, w385) -> (w380:T10[])
            n144 = call <vilib>:"WritePanelData.vi"("error in (no error)"=w381, "Panel Data Array"=w380, "MAUI in"=w383) -> ("error out"=w379:errorcluster, "MAUI out"=w382:refnum<class "SMO.UI.MAUI.Basic.lvclass">)  [unwired: 7 in]
            n145 = Bundle By Name(cluster=w392, "Self Reference"=w382) -> (w391:T5)
            n146 = call <vilib>:"Add State(s) to Queue__jki_lib_state_machine.vi"("State(s) in (\"\")"=w395) -> ("States Out"=w394:string)  [unwired: 14 in]
          }
          frame "MAUI: UpdatePanel" {
            n147 = Decimal String To Number(string=w402) -> (number=w397:i32)  [unwired: 2 in, 1 out]
            n148 = Unbundle By Name(w404) -> ("Self Reference"=w398:refnum<class "SMO.UI.MAUI.Basic.lvclass">, "MAUI.Active Index"=w396:i32)
            n149 = call <vilib>:"SMO.UI.MAUI.UpdatePanel.vi"("error in (no error)"=w401, "Embedded"=w396, "Panel"=w397, "MAUI"=w398) -> ("error out"=w400:errorcluster, "MAUI out"=w399:refnum<class "SMO.UI.MAUI.Basic.lvclass">)  [unwired: 6 in]
            n150 = Bundle By Name(cluster=w404, "Self Reference"=w399) -> (w403:T5)
            n151 = call <vilib>:"Add State(s) to Queue__jki_lib_state_machine.vi"("State(s) in (\"\")"=w407) -> ("States Out"=w406:string)  [unwired: 14 in]
          }
        }
      }
    }
    frame Error {
    }
  }
  n152 = call-parent "Process.vi"("error in"=w7, "MAUI"=w1) -> ("error out"=w5:errorcluster, "MAUI out"=→"MauiTemplate out":refnum<class "SMO.UI.MAUI.Basic.lvclass">)  [unwired: 8 in]
  n153 = Merge Errors(w5, w4) -> (→"error out":errorcluster)
